vi "Read Results from processing.vi"(8 "error in":errorcluster, 11 "Convert Bool to Velocity runtime in":refnum<class "Convert Bool to Velocity runtime.lvclass">) -> (0 "error out":errorcluster, 2 "Results from processing":T1, 3 "Convert Bool to Velocity runtime out":refnum<class "Convert Bool to Velocity runtime.lvclass">)   [LabVIEW 2017, in "Convert Bool to Velocity runtime.lvclass"]
uses:
  Convert Bool to Velocity runtime.lvclass
  configuration/result data indices.ctl
  Convert Bool to Velocity runtime.lvclass/Convert Bool to Velocity runtime.ctl
  configuration/Convert Bool to Velocity configuration.lvclass
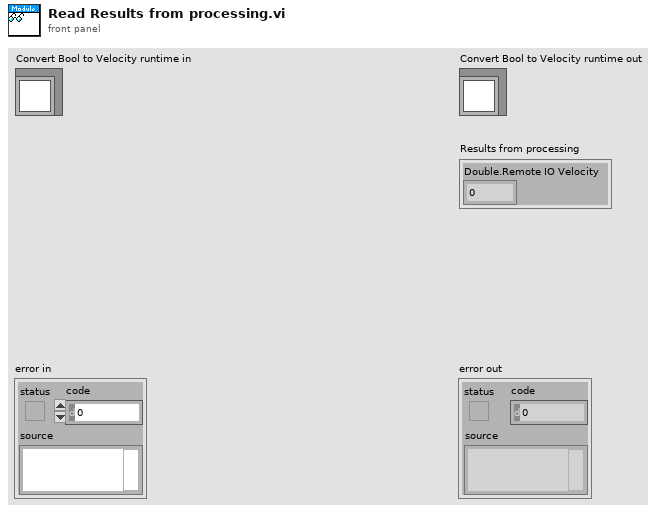
[diagram p1: front panel]
types:
  T1 = typedef "Convert Bool to Velocity configuration.lvclass/result data indices.ctl" = cluster{"Double.Remote IO Velocity":i32}
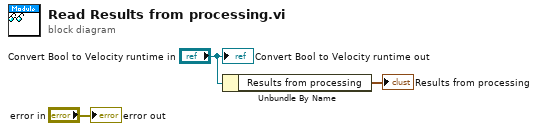
[diagram p0: block diagram]
diagram:
  n1 = Unbundle By Name("Convert Bool to Velocity runtime in") -> ("Results from processing"=→"Results from processing":T1)
  "error out" <- "error in"
  "Convert Bool to Velocity runtime out" <- "Convert Bool to Velocity runtime in"
